vi "Homography_old.vi"() -> ()   [LabVIEW 2015]
uses:
  <vilib>/Analysis/Matrix/Datatypes/RealMatrix.ctl
  <vilib>/Analysis/baseanly.llb/Real A x B.vi
  <vilib>/Analysis/Matrix/Numeric/Conversions/Matrix To Array - RM.vi
  <vilib>/Analysis/baseanly.llb/Real Inverse Matrix.vi
  <vilib>/Analysis/Matrix/Numeric/Conversions/Array To Matrix - RA2.vi
  <vilib>/Analysis/Matrix/Numeric/Multiply/Multiply - RM,RM.vi
  CalibrationCoordinates.vi
  <vilib>/Analysis/Matrix/NI_Matrix.lvlib
  <vilib>/Analysis/NI_AALBase.lvlib
panel:
  out "output array":dbl[](array[numeric])
  out "A x B":T1
  out "XY Graph":cluster{dbl, dbl}[](graph)
  out "appended array":T1
  out "C":T1
  out "B":T1
  out "Image Factors":T1
  out "Image Inverse Matrix":T1
  out "Column":T1
  out "temp":T1
  out "Input":T1
  in  "y":dbl[][](array[numeric])
  in  "x":dbl[][](array[numeric])
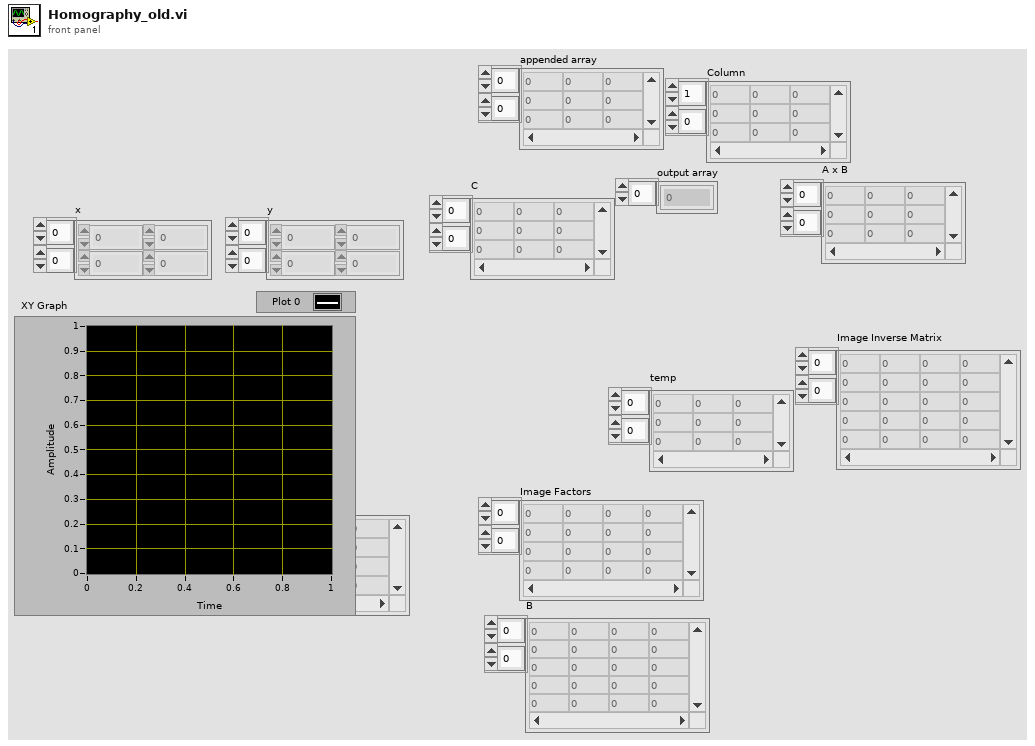
[diagram p1: front panel]
types:
  T1 = typedef "NI_Matrix.lvlib/RealMatrix.ctl" = dbl[][]
  T2 = cluster{"Top Left":dbl[], "Top Right":dbl[], "Bottom Left":dbl[], "Bottom Right":dbl[]}
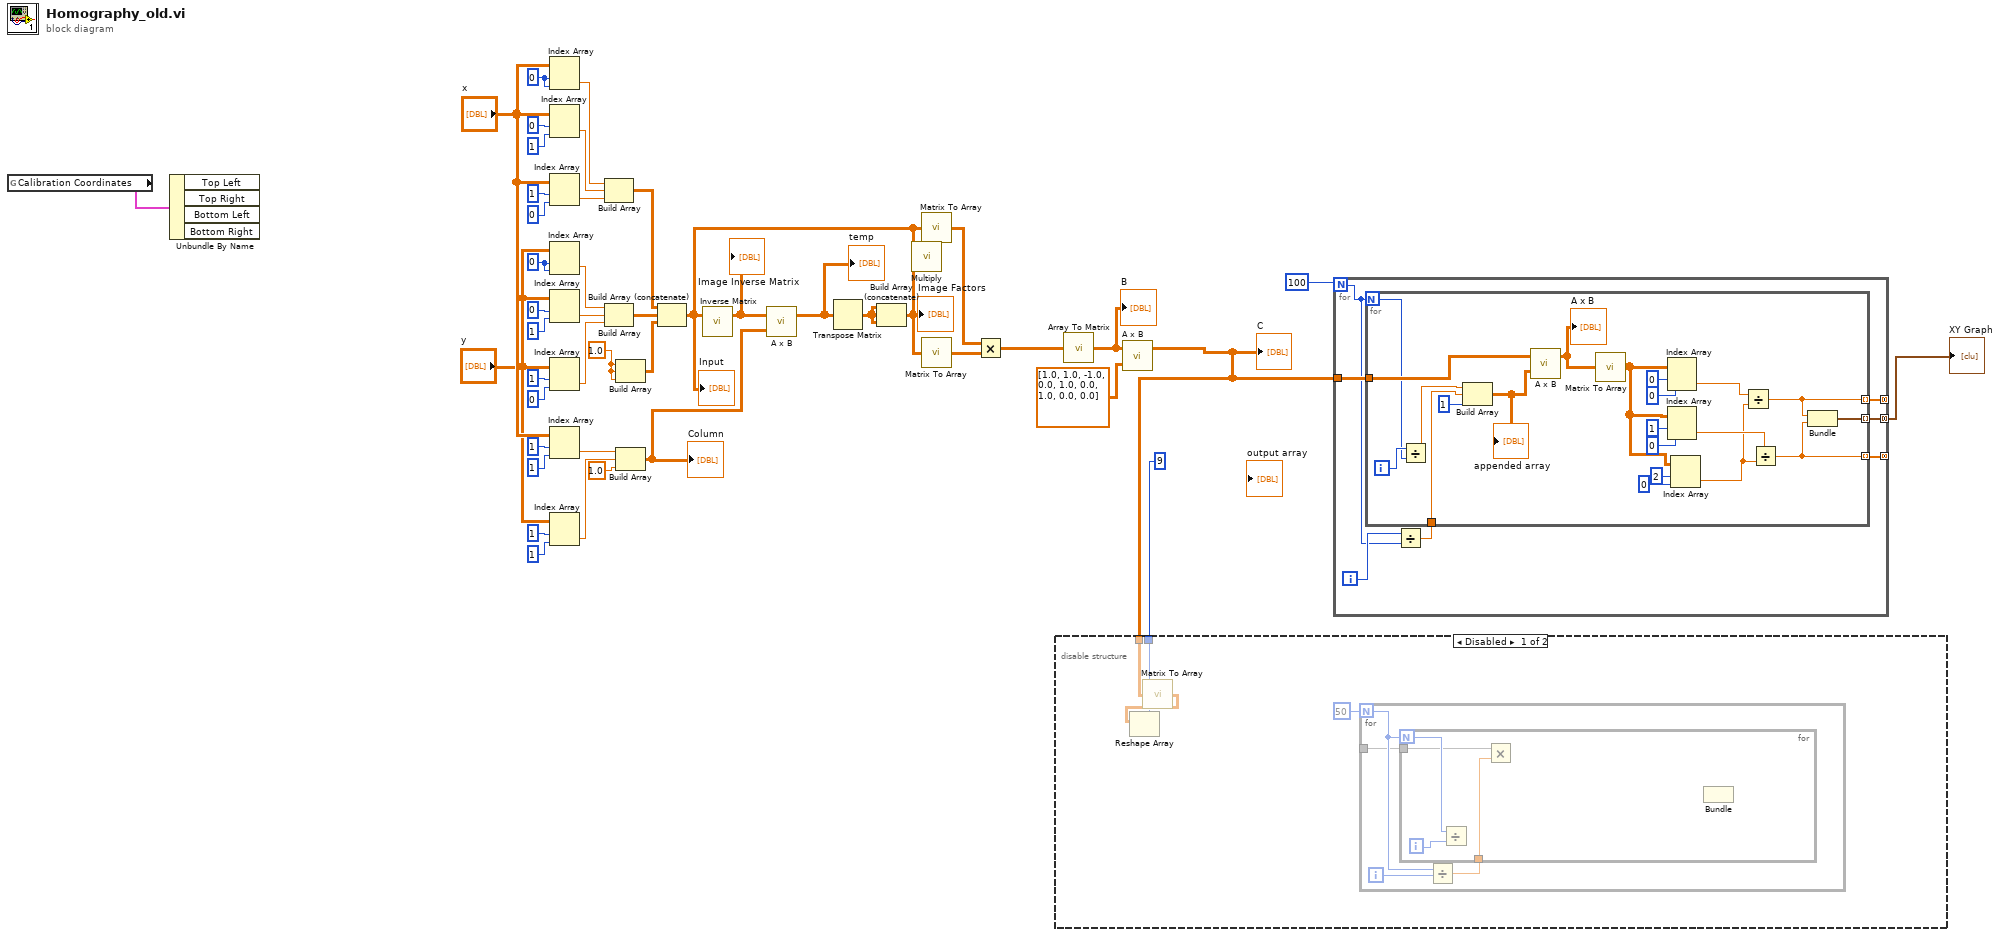
[diagram p0: block diagram]
diagram:
  w31 = 1.0 ("index (row)")
  w35 = 0 ("index (row)")
  w44 = 0 ("index (row)")
  n1 = global read "CalibrationCoordinates.vi" "Calibration Coordinates"() -> (w1:T2)
  n2 = Unbundle By Name(w1) -> ()  [unwired: 4 out]
  n3 = Index Array(array="x", index (row)=w44, index (col)=w44) -> (element=w45:dbl)
  n4 = Index Array(array="x", index (row)=0 ("index (col)"), index (col)=1) -> (element=w40:dbl)
  n5 = Index Array(array="x", index (row)=1, index (col)=0) -> (element=w39:dbl)
  n6 = Index Array(array="y", index (row)=w35, index (col)=w35) -> (element=w32:dbl)
  n7 = Index Array(array="y", index (row)=0 ("index (col)"), index (col)=1) -> (element=w33:dbl)
  n8 = Index Array(array="y", index (row)=1, index (col)=0) -> (element=w34:dbl)
  n9 = Index Array(array="x", index (row)=1, index (col)=1) -> (element=w21:dbl)
  n10 = Index Array(array="y", index (row)=1, index (col)=1) -> (element=w20:dbl)
  n11 = Build Array(w45, w40, w39) -> (w30:T1)
  n12 = Build Array(w32, w33, w34) -> (w29:T1)
  n13 = Build Array(w31, w31, w31) -> (w28:T1)
  n14 = Build Array(w21, w20, 1.0 ("index (row)")) -> (w18:T1)
  "Column" <- w18
  n15 = Build Array (concatenate)(w30, w29, w28) -> (w12:T1)
  "Input" <- w12
  n16 = call-poly <vilib>:"Inverse Matrix.vi"("Input Matrix"=w12) -> ("Inverse Matrix"=w13:T1)  [unwired: 1 in, 1 out]
  "Image Inverse Matrix" <- w13
  n17 = call-poly <vilib>:"A x B.vi"("B"=w18, "A"=w13) -> ("A x B"=w15:T1)  [unwired: 1 out]
  "temp" <- w15
  n18 = Transpose Matrix(1:w15) -> (0:w14:T1)
  n19 = Build Array (concatenate)(w14, w14, w14) -> (w8:T1)
  "Image Factors" <- w8
  n20 = call-poly <vilib>:"Multiply.vi"("Real Matrix B"=w8, "Real Matrix A"=w12) -> ()  [unwired: 1 out]
  n21 = call-poly <vilib>:"Matrix To Array.vi"("Real Matrix"=w12) -> ("Real 2D Array"=w11:dbl[][])
  n22 = call-poly <vilib>:"Matrix To Array.vi"("Real Matrix"=w8) -> ("Real 2D Array"=w9:dbl[][])
  n23 = Multiply(x=w11, y=w9) -> (x*y=w10:dbl[][])
  n24 = call-poly <vilib>:"Array To Matrix.vi"("Real 2D Array"=w10) -> ("Real Matrix"=w7:T1)
  "B" <- w7
  n25 = call-poly <vilib>:"A x B.vi"("B"=T1 [[1.0, 1.0, -1.0], [0.0, 1.0, 0.0], [1.0, 0.0, 0.0]] ("appended array"), "A"=w7) -> ("A x B"=w3:T1)  [unwired: 1 out]
  "C" <- w3
  n26 = disable-structure shown="Disabled" {
    disable-tunnel: w3 -> [w51 _]
    disable-tunnel: 9 ("dimension size") -> [w49 _]
    frame Disabled {
      n27 = call-poly <vilib>:"Matrix To Array.vi"("Real Matrix"=w51) -> ("Real 2D Array"=w50:dbl[][])
      n28 = Reshape Array(w50, w49) -> (w48:dbl[])
      n29 = for {
        N: 50 -> [w54]
        tunnel: [w53] -> w46
        i -> [w55]
        n30 = Divide(x=w54, y=w55) -> (x/y=w52:dbl)
        n31 = for {
          N: w54 -> [w58]
          tunnel: w53 -> [w57]
          tunnel: w52 -> [w56]
          i -> [w59]
          n32 = Divide(x=w58, y=w59) -> ()  [unwired: 1 out]
          n33 = Multiply(x=w57, y=w56) -> ()  [unwired: 1 out]
          n34 = Bundle() -> ()  [unwired: 3 in, 1 out]
        }
      }
    }
    frame Enabled {
    }
  }
  n35 = for {
    N: 100 ("y") -> [w62]
    tunnel: w3 -> [w66]
    tunnel: [w63] -> w4 mode=concatenating
    tunnel: [w61] -> _ mode=concatenating
    tunnel: [w60] -> _ mode=concatenating
    i -> [w65]
    n36 = Divide(x=w65, y=w62) -> (x/y=w64:dbl)
    n37 = for {
      N: w62 -> [w69]
      tunnel: w66 -> [w82]
      tunnel: w64 -> [w85]
      tunnel: [w70] -> w63 mode=indexing
      tunnel: [w68] -> w61 mode=indexing
      tunnel: [w67] -> w60 mode=indexing
      i -> [w86]
      n38 = Divide(x=w86, y=w69) -> (x/y=w84:dbl)
      n39 = Build Array(w84, w85, 1 ("index (row)")) -> (w83:T1)
      "appended array" <- w83
      n40 = call-poly <vilib>:"A x B.vi"("B"=w83, "A"=w82) -> ("A x B"=w81:T1)  [unwired: 1 out]
      "A x B" <- w81
      n41 = call-poly <vilib>:"Matrix To Array.vi"("Real Matrix"=w81) -> ("Real 2D Array"=w77:dbl[][])
      n42 = Index Array(array=w77, index (row)=0, index (col)=0 ("disabled index (col)")) -> (element=w73:dbl)
      n43 = Index Array(array=w77, index (row)=1, index (col)=0 ("disabled index (col)")) -> (element=w72:dbl)
      n44 = Index Array(array=w77, index (row)=2, index (col)=0 ("disabled index (col)")) -> (element=w71:dbl)
      n45 = Divide(x=w73, y=w71) -> (x/y=w67:dbl)
      n46 = Divide(x=w72, y=w71) -> (x/y=w68:dbl)
      n47 = Bundle(w67, w68) -> (w70:cluster{dbl, dbl})  [unwired: 1 in]
    }
  }
  "XY Graph" <- w4
